vi "main.vi"() -> ()   [LabVIEW 2018]
panel:
  out "Sol":i32
  out "high/lower peak":dbl[][](array[numeric])
  out "斜率":dbl[][](array[numeric])
  out "Array":i32[](array[numeric])
  out "有n!組排列組合":i32[](array[numeric])
  out "排列組合":i32[][](array[numeric])
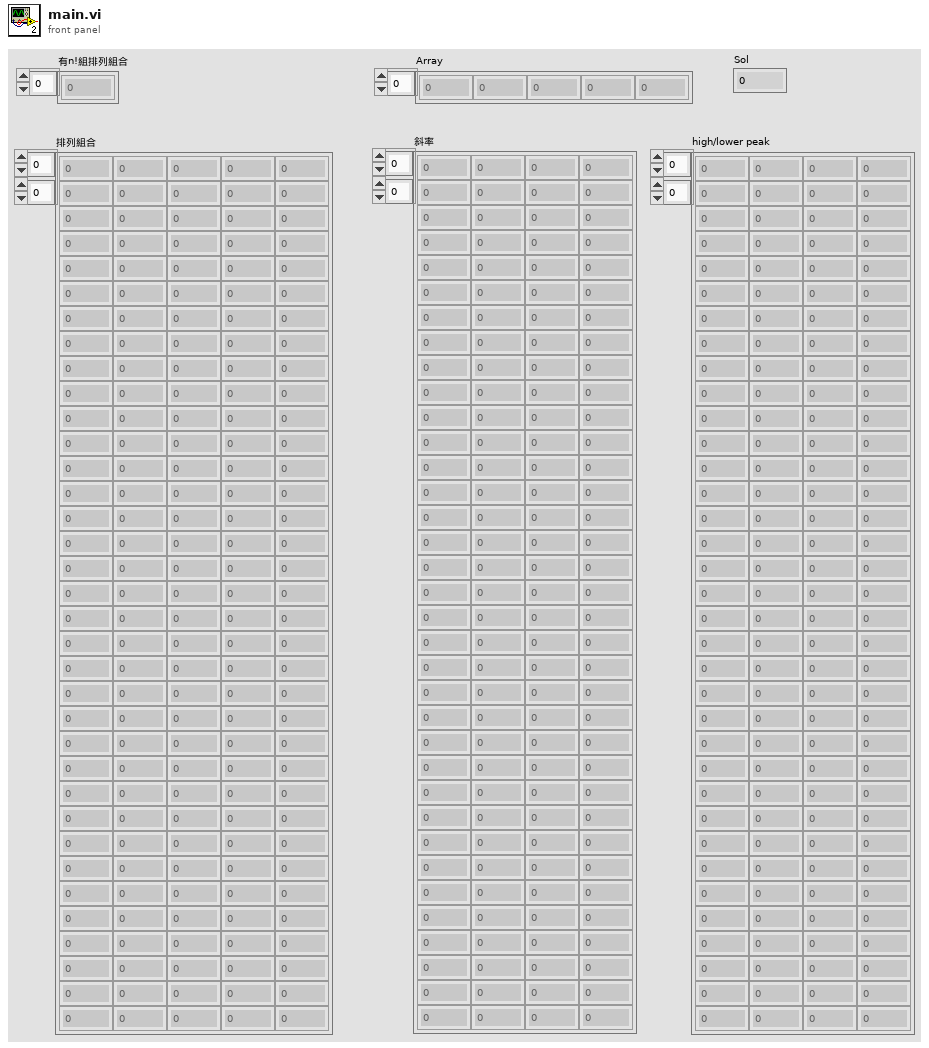
[diagram p1: front panel]
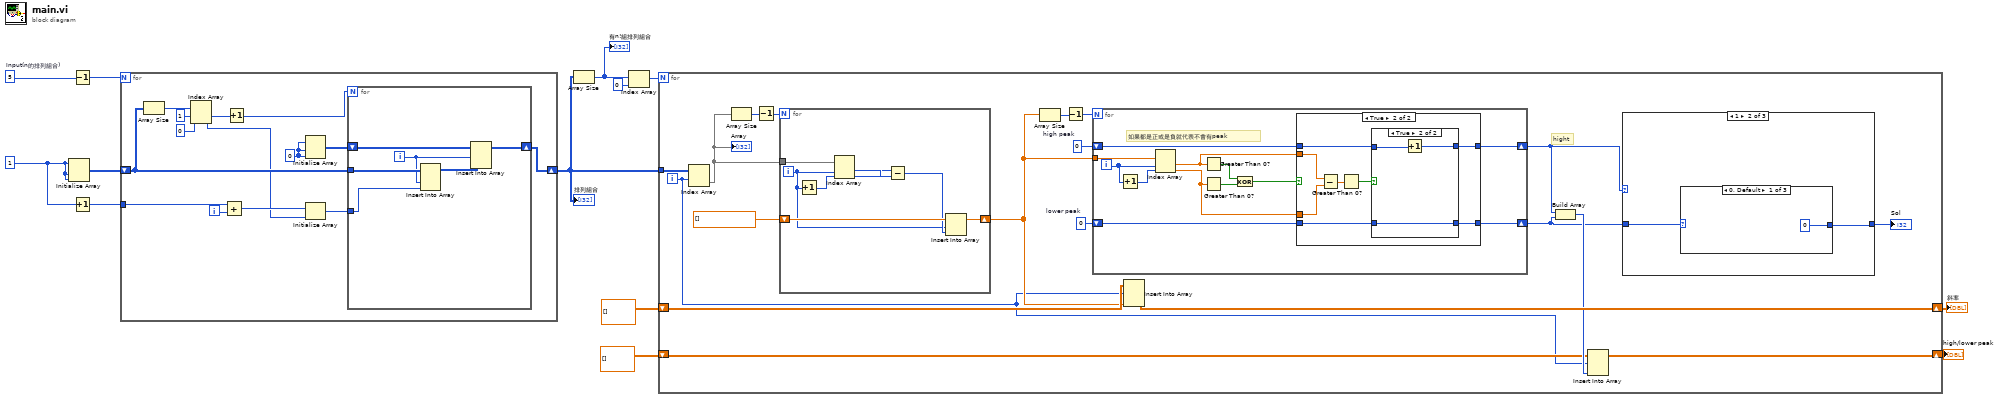
[diagram p0: block diagram]
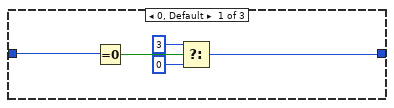
[diagram p2: hidden frame]
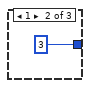
[diagram p3: hidden frame]
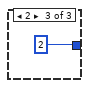
[diagram p4: hidden frame]
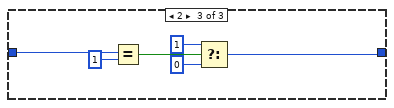
[diagram p5: hidden frame]
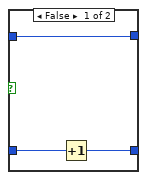
[diagram p7: hidden frame]
diagram:
  w5 = 5  # Input(n的排列組合)
  w6 = 1
  n1 = Initialize Array(w6, w6, w6) -> (w12:i32[][])
  n2 = Decrement(x=w5) -> (x-1=w13:i32)
  n3 = Increment(x=w6) -> (x+1=w11:i32)
  n4 = for {
    N: w13 -> [_]
    tunnel: w11 -> [w19]
    shift-right: [w15] -> w7
    shift-left: w12 -> [w20]
    i -> [w14]
    w21 = 0 ("dimension size")
    n5 = Array Size(array=w20) -> (size(s)=w26:i32[])
    n6 = Index Array(array=w26, index #1=1 ("index (row)"), index #2=0 ("disabled index (col)")) -> (element #1=w24:i32, element #2=w17:i32)
    n7 = Add(x=w19, y=w14) -> (x+y=w18:i32)
    n8 = Increment(x=w24) -> (x+1=w23:i32)
    n9 = Initialize Array(w21, w21, w21) -> (w22:i32[][])
    n10 = Initialize Array(w18, w17) -> (w16:i32[])
    n11 = for {
      N: w23 -> [_]
      tunnel: w20 -> [w31]
      shift-right: [w33] -> w15
      shift-left: w22 -> [w32]
      tunnel: w16 -> [w30]
      i -> [w29]
      n12 = Insert Into Array(array=w31, index (col)=w29, new element=w30) -> (w28:i32[][])  [unwired: 1 in]
      n13 = Insert Into Array(array=w32, index (row)=w29, new element=w28) -> (w33:i32[][])  [unwired: 1 in]
    }
  }
  "排列組合" <- w7
  n14 = Array Size(array=w7) -> (size(s)=w10:i32[])
  "有n!組排列組合" <- w10
  n15 = Index Array(array=w10, index=0) -> (element=w8:i32)
  n16 = for {
    N: w8 -> [_]
    tunnel: w7 -> [w52]
    shift-right: [w46] -> w3
    shift-left: dbl[][] [] -> [w47]
    shift-right: [w37] -> w1
    shift-left: dbl[][] [] -> [w39]
    i -> [w38]
    w41 = 0  # lower peak
    w42 = 0  # high peak
    # "hight"
    n17 = Index Array(array=w52, index (row)=w38) -> (element=w51:i32[])  [unwired: 1 in]
    "Array" <- w51
    n18 = Array Size(array=w51) -> (size(s)=w48:i32)
    n19 = Decrement(x=w48) -> (x-1=w50:i32)
    n20 = for {
      N: w50 -> [_]
      tunnel: w51 -> [w104]
      shift-right: [w98] -> w43
      shift-left: dbl[] [] -> [w102]
      i -> [w97]
      n21 = Increment(x=w97) -> (x+1=w103:i32)
      n22 = Index Array(array=w104, index #1=w97, index #2=w103) -> (element #1=w101:i32, element #2=w100:i32)
      n23 = Subtract(x=w100, y=w101) -> (x-y=w99:i32)
      n24 = Insert Into Array(array=w102, index=w97, new element=w99) -> (w98:dbl[])
    }
    n25 = Array Size(array=w43) -> (size(s)=w45:i32)
    n26 = Decrement(x=w45) -> (x-1=w44:i32)
    n27 = for {
      N: w44 -> [_]
      tunnel: w43 -> [w78]
      shift-right: [w74] -> w36
      shift-left: w42 -> [w77]
      shift-right: [w75] -> w35
      shift-left: w41 -> [w76]
      i -> [w79]
      # "如果都是正或是負就代表不會有peak"
      n28 = Increment(x=w79) -> (x+1=w80:i32)
      n29 = Index Array(array=w78, index #1=w79, index #2=w80) -> (element #1=w72:dbl, element #2=w71:dbl)
      n30 = Greater Than 0?(x=w72) -> (x > 0?=w73:bool)
      n31 = Greater Than 0?(x=w71) -> (x > 0?=w69:bool)
      n32 = Exclusive Or(1:w69, 2:w73) -> (0:w70:bool)
      n33 = case shown="True" w70 {
        tunnel: w77 -> [w82 w88]
        tunnel: w76 -> [w81 w87]
        tunnel: [w81 w86] -> w75
        tunnel: [w82 w85] -> w74
        tunnel: w72 -> [_ w83]
        tunnel: w71 -> [_ w84]
        frame False {
        }
        frame True {
          n34 = Subtract(x=w83, y=w84) -> (x-y=w89:dbl)
          n35 = Greater Than 0?(x=w89) -> (x > 0?=w90:bool)
          n36 = case shown="True" w90 {
            tunnel: w88 -> [w93 w96]
            tunnel: w87 -> [w92 w95]
            tunnel: [w93 w94] -> w85
            tunnel: [w91 w95] -> w86
            frame False {
              n37 = Increment(x=w92) -> (x+1=w91:i32)
            }
            frame True {
              n38 = Increment(x=w96) -> (x+1=w94:i32)
            }
          }
        }
      }
    }
    n39 = Insert Into Array(array=w47, index (row)=w38, new element=w43) -> (w46:dbl[][])  [unwired: 1 in]
    n40 = Build Array(w36, w35) -> (w40:i32[])
    n41 = Insert Into Array(array=w39, index (row)=w38, new element=w40) -> (w37:dbl[][])  [unwired: 1 in]
    n42 = case shown="1" w36 {
      tunnel: w35 -> [w57 w59 w63]
      tunnel: [w53 w58 w64] -> w34
      frame 0, Default {
        n43 = Equal To 0?(x=w57) -> (x = 0?=w56:bool)
        n44 = Select(t=3, s=w56, f=0) -> (s? t:f=w53:i32)
      }
      frame 1 {
        n45 = case shown="0, Default" w59 {
          tunnel: [0 ("y") 3 ("y") 2 ("y")] -> w58
          frame 0, Default {
          }
          frame 1 {
          }
          frame 2 {
          }
        }
      }
      frame 2 {
        n46 = Equal?(x=w63, y=1) -> (x = y?=w68:bool)
        n47 = Select(t=1, s=w68, f=0) -> (s? t:f=w64:i32)
      }
    }
    "Sol" <- w34
  }
  "斜率" <- w3
  "high/lower peak" <- w1
